vi "Mouse Wait Ready.vi"(2 "Timeout (ms)":i32, 3 "Refnum in":refnum<k20>) -> (0 "Timeout":bool, 1 "Refnum out":refnum<k20>)   [LabVIEW 2012]
uses:
  <vilib>/Utility/error.llb/Error Cluster From Error Code.vi
  <vilib>/rvi/errors/niLvFpgaAdjustHostInterfaceError.vi
  <vilib>/rvi/interface/nirviReadWriteControl/nirviReadWriteControl.xnode
  NiFpgaLv.dll
  <vilib>/rvi/interface/Simulation/niFpgaSimulationCallBeginRW.vi
panel:
  # "DESC\n=====\nWaits for FPGA Mouse IO state machinetosignal that it has\nfinished the previous opperation."
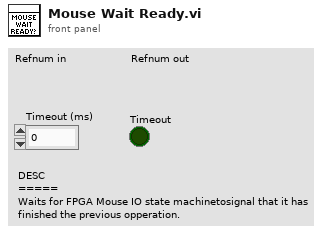
[diagram p1: front panel]
types:
  T1 = enum16{"idle", "set idle", "begin", "write", "read", "power down", "reset"}
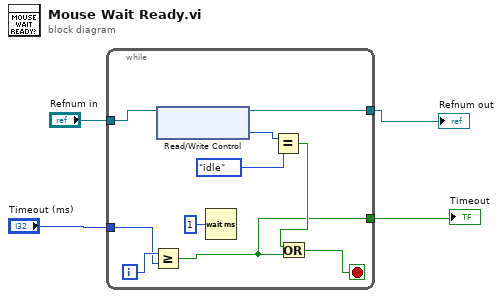
[diagram p0: block diagram]
diagram:
  n1 = while {
    tunnel: "Refnum in" -> [w14]
    tunnel: [w8] -> w3
    tunnel: "Timeout (ms)" -> [w5]
    tunnel: [w7] -> w1
    i -> [w6]
    stop <- w9 stop-if-true
    n2 = Greater Or Equal?(x=w6, y=w5) -> (x >= y?=w7:bool)
    n3 = xnode "Read/Write Control"("FPGA VI Reference In"=w14) -> ("FPGA VI Reference Out"=w8:refnum<k20>, "Mouse Action"=w13:T1)  [unwired: 1 in, 1 out]
    n4 = Wait (ms)(milliseconds to wait=u32 1) -> ()  [unwired: 1 out]
    n5 = Equal?(x=w13, y=T1."idle") -> (x = y?=w10:bool)
    n6 = Or(x=w10, y=w7) -> (x .or. y?=w9:bool)
  }
  "Refnum out" <- w3
  "Timeout" <- w1
